vi "FisherPaykel Check Motor Profile Status.vi"(8 "Error In":errorcluster, 11 "ERD Array":string[][](array[string])=[["Motor Profile Status (0xF0B7)", "Started"], ["Motor Profile (0xF0B7)", "9"], ["Motor Mode (0xF0B1)", "Idle"], ["Mode Shift Status (0xFF22)", "Agitate State"], ["Sub-Cycle (0xF07B)", "WASH"], ["Remaining Cycle Time(s) (0xF061)", "1707"], ["Target Speed (RPM) (0xF0AC)", "0"]]) -> (0 "Error Out":errorcluster, 2 "Motor Profile Data":T1, 3 "States Output":string)   [LabVIEW 2016]
uses:
  Type Definitions/FisherPaykel Motor Profile Data ERD.ctl
panel:
  # "The first check is too see if the motor should be running."
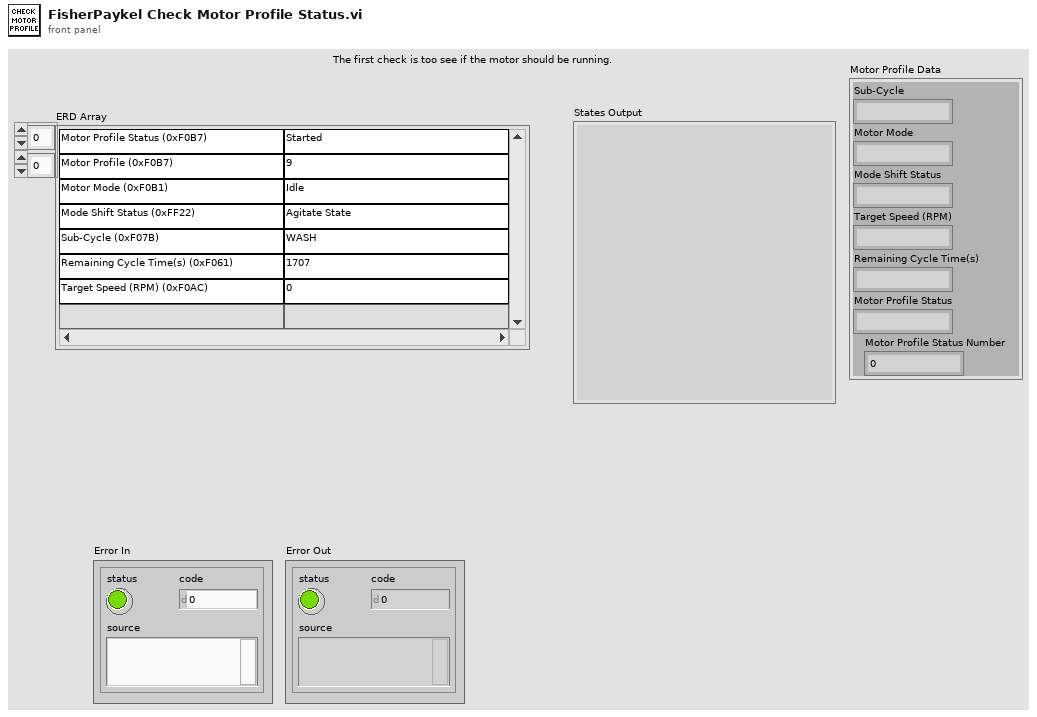
[diagram p1: front panel]
types:
  T1 = typedef "FisherPaykel Motor Profile Data ERD.ctl" = cluster{"Sub-Cycle":string, "Motor Mode":string, "Mode Shift Status":string, "Target Speed (RPM)":string, "Remaining Cycle Time(s)":string, "Motor Profile Status":string, "Motor Profile Status Number":u16}
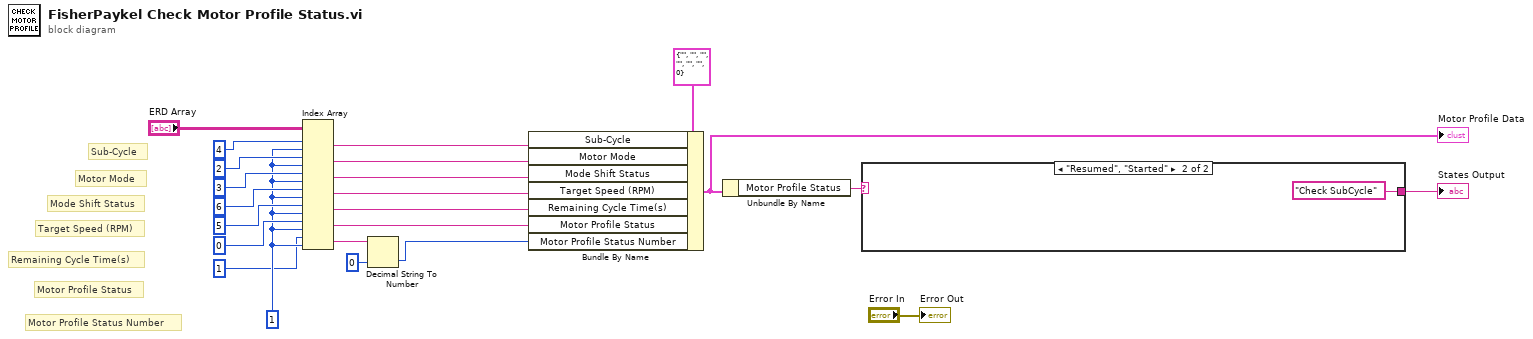
[diagram p0: block diagram]
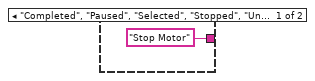
[diagram p2: hidden frame]
diagram:
  w5 = 1 ("disabled index (col)")
  # "Motor Profile Status Number"
  # "Motor Profile Status"
  # "Remaining Cycle Time(s)"
  # "Target Speed (RPM)"
  # "Sub-Cycle"
  # "Mode Shift Status"
  # "Motor Mode"
  n1 = Index Array(array="ERD Array", index (row) #1=4 ("disabled index (row)"), index (col) #1=w5, index (row) #2=2 ("disabled index (row)"), index (col) #2=w5, index (row) #3=3 ("disabled index (row)"), index (col) #3=w5, index (row) #4=6 ("disabled index (row)"), index (col) #4=w5, index (row) #5=5 ("disabled index (row)"), index (col) #5=w5, index (row) #6=0 ("disabled index (row)"), index (col) #6=w5, index (row) #7=1 ("disabled index (row)"), index (col) #7=w5) -> (element #1=w13:string, element #2=w12:string, element #3=w11:string, element #4=w10:string, element #5=w9:string, element #6=w8:string, element #7=w3:string)
  n2 = Decimal String To Number(string=w3, default (0L)=u16 0 ("default (0 I32)")) -> (number=w2:u16)  [unwired: 1 in, 1 out]
  n3 = Bundle By Name(cluster=T1 {"Sub-Cycle"="", "Motor Mode"="", "Mode Shift Status"="", "Target Speed (RPM)"="", "Remaining Cycle Time(s)"="", "Motor Profile Status"="", "Motor Profile Status Number"=0}, "Sub-Cycle"=w13, "Motor Mode"=w12, "Mode Shift Status"=w11, "Target Speed (RPM)"=w10, "Remaining Cycle Time(s)"=w9, "Motor Profile Status"=w8, "Motor Profile Status Number"=w2) -> (w7:T1)
  "Motor Profile Data" <- w7
  n4 = Unbundle By Name(w7) -> ("Motor Profile Status"=w6:string)
  n5 = case shown="\"Resumed\", \"Started\"" w6 {
    tunnel: ["Stop Motor" ("States Output") "Check SubCycle" ("States Output")] -> w23
    frame "Completed", "Paused", "Selected", "Stopped", "Unknown", Default {
    }
    frame "Resumed", "Started" {
    }
  }
  "States Output" <- w23
  "Error Out" <- "Error In"
